vi "ArrayS2ArrayAx_.vi"(3 "Signal_input":string, 4 "Signals_value_Array":sgl[](array[numeric]), 5 "Signals_name":string[](array[string])) -> (0 "Subarray 1x_out":sgl[](array[numeric]), 1 "Subarray 2x_out":sgl[][](array[numeric]), 2 "Signal out":string)   [LabVIEW 2021]
doc: "This function converts an array of strings into an array of arrays of numeric values."
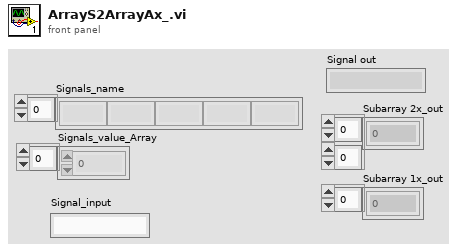
[diagram p1: front panel]
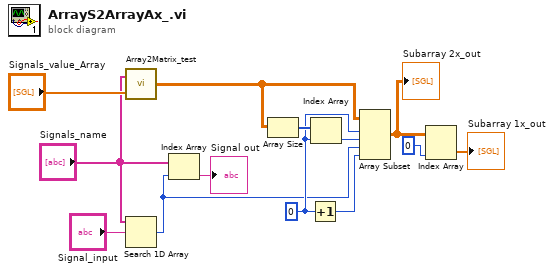
[diagram p0: block diagram]
diagram:
  w9 = 0 ("index")
  n1 = call "Array2Matrix_test.vi"("Array"="Signals_value_Array", "Header"="Signals_name") -> ("Array2D"=w12:sgl[][])
  n2 = Search 1D Array(1D array="Signals_name", element="Signal_input") -> (index of element=w2:i32)  [unwired: 1 in]
  n3 = Index Array(array="Signals_name", index=w2) -> (element=→"Signal out":string)
  n4 = Array Size(array=w12) -> (size(s)=w11:i32[])
  n5 = Increment(x=w9) -> (x+1=w8:i32)
  n6 = Index Array(array=w11, index=w9) -> (element=w10:i32)
  n7 = Array Subset(array=w12, index (row)=w9, length (row)=w10, index (col)=w2, length (col)=w8) -> (w7:sgl[][])
  "Subarray 2x_out" <- w7
  n8 = Index Array(array=w7, index (col)=0 ("disabled index (col)")) -> (element=→"Subarray 1x_out":sgl[])  [unwired: 1 in]
